vi "spring - update itemstrings.vi"(7 "tree ref":refnum<vi>, 8 "error in (no error)":errorcluster, 10 "itemstrings":string[](array[string]), 11 "node data":T1) -> (0 "error out":errorcluster, 3 "node data out":T1)   [LabVIEW 2014]
uses:
  spring - node data.ctl
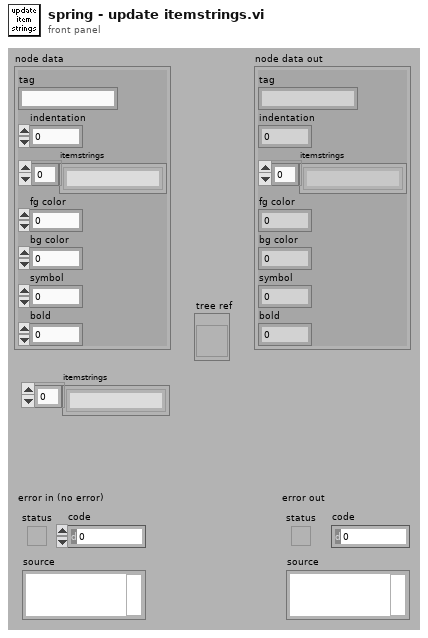
[diagram p1: front panel]
types:
  T1 = typedef "spring - node data.ctl" = cluster{"tag":string, "indentation":i32, "itemstrings":string[], "fg color":u32, "bg color":u32, "symbol":u32, "bold":u32}
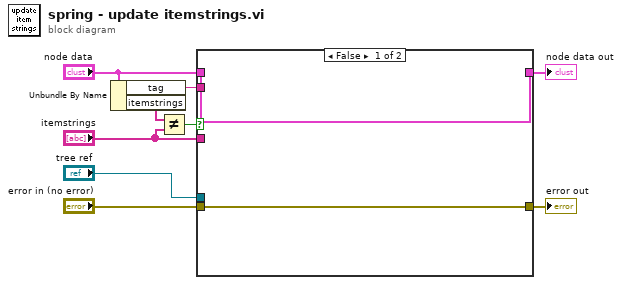
[diagram p0: block diagram]
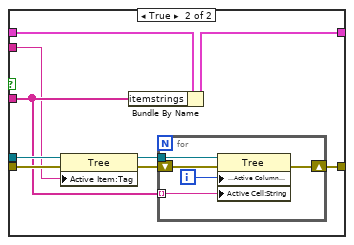
[diagram p2: hidden frame]
diagram:
  n1 = Unbundle By Name("node data") -> ("tag"=w1:string, "itemstrings"=w4:string[])
  n2 = Not Equal?(x=w4, y="itemstrings") -> (x != y?=w2:bool)
  n3 = case shown="False" w2 {
    tunnel: "error in (no error)" -> [w10 w19]
    tunnel: "tree ref" -> [_ w17]
    tunnel: [w10 w16] -> w7
    tunnel: [w11 w15] -> w6
    tunnel: "node data" -> [w11 w13]
    tunnel: "itemstrings" -> [_ w14]
    tunnel: w1 -> [_ w12]
    frame False {
    }
    frame True {
      n4 = property on="Property Node" class="Tree"(reference=w17, error in=w19, "Active Item:Tag"=w12) -> (reference out=w18:refnum<vi>, error out=w20:errorcluster)
      n5 = Bundle By Name(cluster=w13, "itemstrings"=w14) -> (w15:T1)
      n6 = for {
        tunnel: w18 -> [w25]
        shift-right: [w22] -> w16
        shift-left: w20 -> [w23]
        tunnel: w14 -> [w21] mode=indexing
        i -> [w24]
        n7 = property on="Property Node" class="Tree"(reference=w25, error in=w23, "Active Cell:Active Column Number"=w24, "Active Cell:String"=w21) -> (error out=w22:errorcluster)  [unwired: 1 out]
      }
    }
  }
  "error out" <- w7
  "node data out" <- w6
